vi "FrontPanel.vi"(8 "error in":errorcluster, 11 "PythonConverter_GUI in":refnum<class "PythonConverter_GUI.lvclass">) -> (0 "error out":errorcluster, 3 "PythonConverter_GUI out":refnum<class "PythonConverter_GUI.lvclass">, 4 "FrontPanel":string)   [LabVIEW 2014, in "PythonConverter_GUI.lvclass"]
uses:
  PythonConverter_GUI.lvclass
  Parsing/Python Functions.lvlib
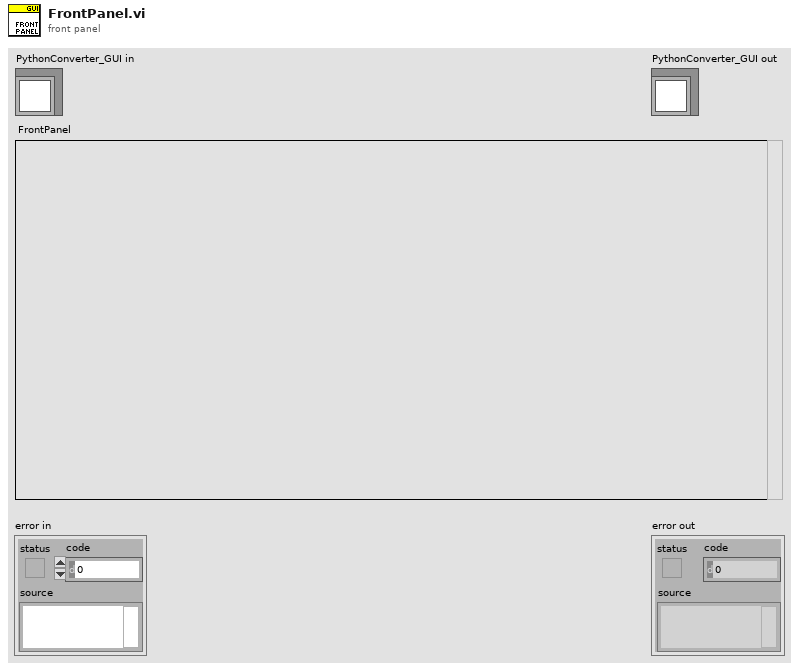
[diagram p1: front panel]
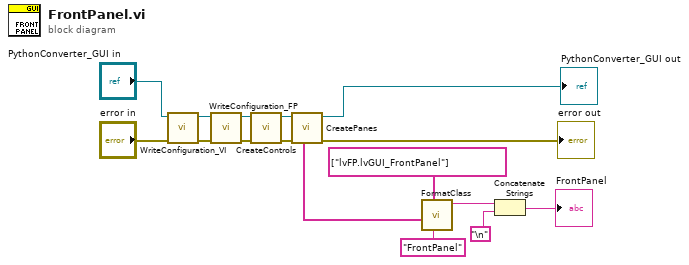
[diagram p0: block diagram]
diagram:
  n1 = call "WriteConfiguration_VI.vi"("error in"="error in", "PythonConverter_GUI in"="PythonConverter_GUI in") -> ("error out"=w3:errorcluster, "PythonConverter_GUI out"=w4:refnum<class "PythonConverter_GUI.lvclass">)  [unwired: 8 in]
  n2 = call "WriteConfiguration_FP.vi"("error in"=w3, "PythonConverter_GUI in"=w4) -> ("error out"=w9:errorcluster, "PythonConverter_GUI out"=w8:refnum<class "PythonConverter_GUI.lvclass">)  [unwired: 8 in]
  n3 = call "CreateControls.vi"("error in"=w9, "PythonConverter_GUI in"=w8) -> ("error out"=w10:errorcluster, "PythonConverter_GUI out"=w7:refnum<class "PythonConverter_GUI.lvclass">)  [unwired: 8 in]
  n4 = call "CreatePanes.vi"("error in"=w10, "PythonConverter_GUI in"=w7) -> ("error out"=→"error out":errorcluster, "PythonConverter_GUI out"=→"PythonConverter_GUI out":refnum<class "PythonConverter_GUI.lvclass">, "panes"=w5:string[])  [unwired: 7 in]
  n5 = call "FormatClass.vi"("name"="FrontPanel", "parameters/ancestors"=string[] ["lvFP.lvGUI_FrontPanel"], "body"=w5) -> ("python"=w13:string)  [unwired: 8 in]
  n6 = Concatenate Strings(w13, "\n") -> (→"FrontPanel":string)
